vi "Withdraw and Check Funds.vi"(10 "Withdraw amount ($)":dbl, 11 "Data Cluster in":T1) -> (0 "error out":errorcluster, 3 "Data Cluster out":T1)   [LabVIEW 2020, in "Money.lvlib"]
uses:
  Money.lvlib
  Module Data--cluster.ctl
  <vilib>/ErrorRing/Error Ring.xnode
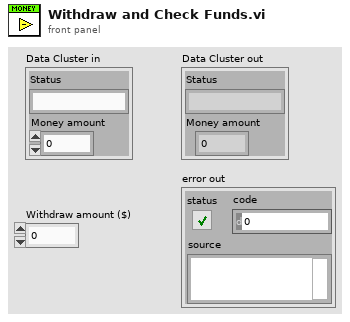
[diagram p1: front panel]
types:
  T1 = typedef "Money.lvlib/Module Data--cluster.ctl" = cluster{"Status":string, "Money amount":dbl}
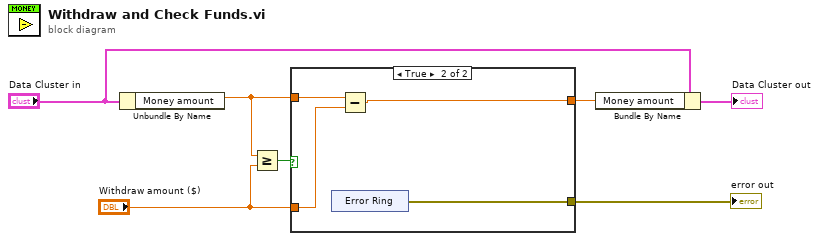
[diagram p0: block diagram]
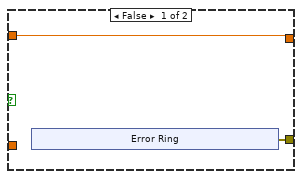
[diagram p2: hidden frame]
diagram:
  n1 = Unbundle By Name("Data Cluster in") -> ("Money amount"=w3:dbl)
  n2 = Greater Or Equal?(x=w3, y="Withdraw amount ($)") -> (x >= y?=w4:bool)
  n3 = case shown="True" w4 {
    tunnel: [w9 w14] -> w7
    tunnel: "Withdraw amount ($)" -> [_ w13]
    tunnel: w3 -> [w9 w12]
    tunnel: [w8 w11] -> w1
    frame False {
      n4 = xnode "Error Ring"() -> ("error out"=w8:errorcluster)
    }
    frame True {
      n5 = xnode "Error Ring"() -> ("error out"=w11:errorcluster)
      n6 = Subtract(x=w12, y=w13) -> (x-y=w14:dbl)
    }
  }
  "error out" <- w1
  n7 = Bundle By Name(cluster="Data Cluster in", "Money amount"=w7) -> (→"Data Cluster out":T1)
